vi "UsrProfiles-Sort profiles names.vi"(11 "User profile names":string[](array[string])) -> (3 "User profile names":string[](array[string]))   [LabVIEW 2017]
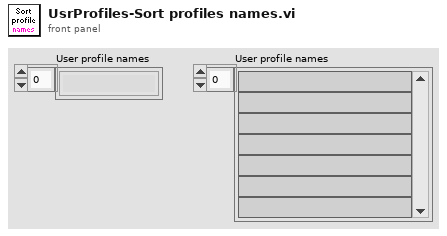
[diagram p1: front panel]
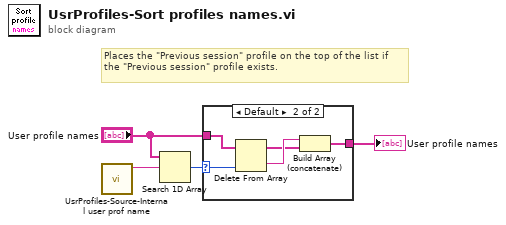
[diagram p0: block diagram]
diagram:
  # "Places the \"Previous session\" profile on the top of the list if the \"Previous session\" profile exists."
  n1 = call "UsrProfiles-Source-Internal user prof name.vi"() -> ("Previous session profile name"=w4:string)  [unwired: 11 in]
  n2 = Search 1D Array(1D array="User profile names", element=w4) -> (index of element=w1:i32)  [unwired: 1 in]
  n3 = case shown="Default" w1 {
    selector: w1 -> [_ w6]
    tunnel: "User profile names" -> [w5 w8]
    tunnel: [w5 w7] -> w2
    frame -1 {
    }
    frame Default {
      n4 = Delete From Array(array=w8, index=w6) -> (deleted portion=w10:string, array with subset deleted=w9:string[])  [unwired: 1 in]
      n5 = Build Array (concatenate)(w10, w9) -> (w7:string[])
    }
  }
  "User profile names" <- w2
